vi "Excelmain.vi"() -> ()   [LabVIEW 2017]
panel:
  out "错误输出":errorcluster
  in  "Filename":string="D:\\\\project.xls" caption="工作簿文件名"
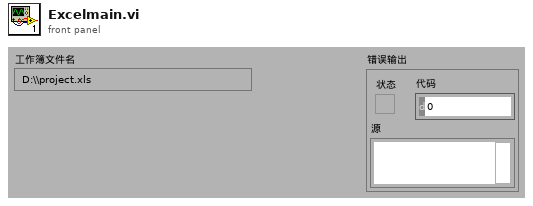
[diagram p1: front panel]
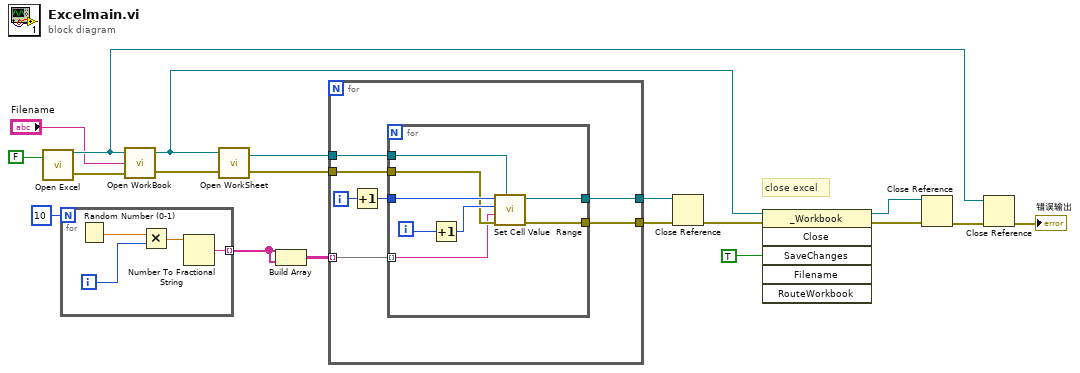
[diagram p0: block diagram]
diagram:
  # "close excel"
  n1 = call "Open Excel.vi"("Visible Boolean"=FALSE) -> ("error out"=w19:errorcluster, "Excel._Application"=w10:refnum<k7>)  [unwired: 1 in]
  n2 = for {
    N: 10 -> [_]
    tunnel: [w20] -> w16 mode=indexing
    i -> [w22]
    n3 = Random Number (0-1)() -> (number: 0 to 1=w23:dbl)
    n4 = Multiply(x=w23, y=w22) -> (x*y=w21:dbl)
    n5 = Number To Fractional String(number=w21) -> (F-format string=w20:string)  [unwired: 3 in]
  }
  n6 = call "Open WorkBook.vi"("error in (no error)"=w19, "Filename of Workbook"="Filename", "Excel._Application"=w10) -> ("error out"=w18:errorcluster, "Excel._Workbook"=w2:refnum<k7>)
  n7 = call "Open WorkSheet.vi"("error in (no error)"=w18, "Excel._Workbook"=w2) -> ("error out"=w14:errorcluster, "Excel._Worksheet"=w15:refnum<k7>)  [unwired: 1 in]
  n8 = Build Array(w16, w16) -> (w13:string[][])
  n9 = for {
    tunnel: w15 -> [w28]
    tunnel: [w27] -> w1
    tunnel: w14 -> [w26]
    tunnel: [w25] -> w12
    tunnel: w13 -> [w24] mode=indexing
    i -> [w30]
    n10 = Increment(x=w30) -> (x+1=w29:i32)
    n11 = for {
      tunnel: w29 -> [w37]
      tunnel: w28 -> [w35]
      tunnel: [w34] -> w27
      tunnel: w26 -> [w33]
      tunnel: [w32] -> w25
      tunnel: w24 -> [w31] mode=indexing
      i -> [w38]
      n12 = Increment(x=w38) -> (x+1=w36:i32)
      n13 = call "Set Cell Value  Range.vi"("Excel._Worksheet"=w35, "error in"=w33, "Value"=w31, "Col"=w36, "Row"=w37) -> ("error out"=w32:errorcluster, "Excel._Worksheet"=w34:refnum<k7>)  [unwired: 2 out]
    }
  }
  n14 = Close Reference(reference=w1, error in (no error)=w12) -> (error out=w7:errorcluster)
  n15 = invoke class="_Workbook" method="Close"(reference=w2, error in=w7, "SaveChanges"=TRUE) -> (reference out=w5:refnum<k7>, error out=w4:errorcluster)  [unwired: 3 in, 4 out]
  n16 = Close Reference(reference=w5, error in (no error)=w4) -> (error out=w11:errorcluster)
  n17 = Close Reference(reference=w10, error in (no error)=w11) -> (error out=→"错误输出":errorcluster)
